vi "FPGA_HoppingStep(NoXYCalculation).vi"() -> ()   [LabVIEW 2014]
uses:
  <vilib>/rvi/Emulation/niFpgaGetClockAttributes.vi
  <vilib>/rvi/Emulation/niFpgaSctlEmulationGetInTimedLoop.vi
  <vilib>/rvi/Emulation/niFpgaEmulationReportErrorSimple.vi
  <vilib>/rvi/interface/RandomDataEmulation/niFpgaRandomDataHandleErrors.vi
  <vilib>/rvi/eio/common/nirviEmuTemplateMethod_errors.vi
  <vilib>/rvi/Emulation/niFpgaProcessEmulError.vi
  <vilib>/rvi/Emulation/niFpgaCriticalErrorInLSC.vi
  <vilib>/rvi/DataTransferAndStorage/Container/XNode/niFpgaContainer.xnode
  <vilib>/rvi/interface/RandomDataEmulation/nirviRandomDataFpgaReadWriteTemplate.vi
  <vilib>/eio/EIONode/EIONode.xnode
panel:
  out "ZPresPos":i16
  in  "stop":bool
  in  "Sleep us":i16
  in  "RelativeWithdraw":i16
  in  "ZOffset":i16
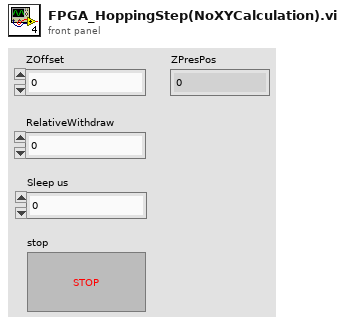
[diagram p1: front panel]
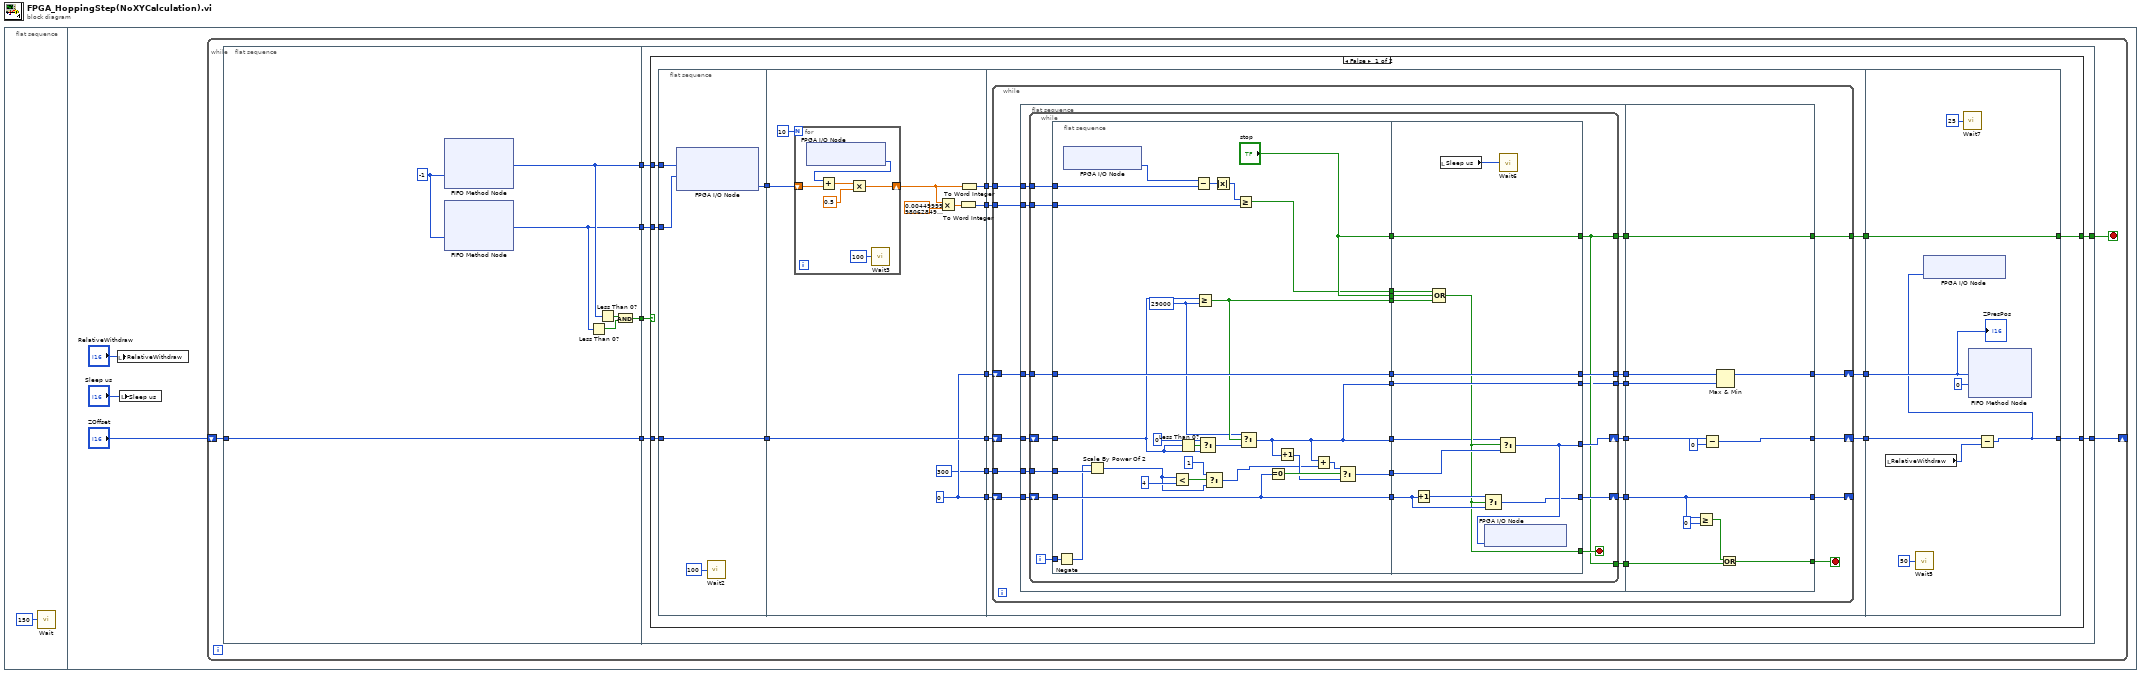
[diagram p0: block diagram]
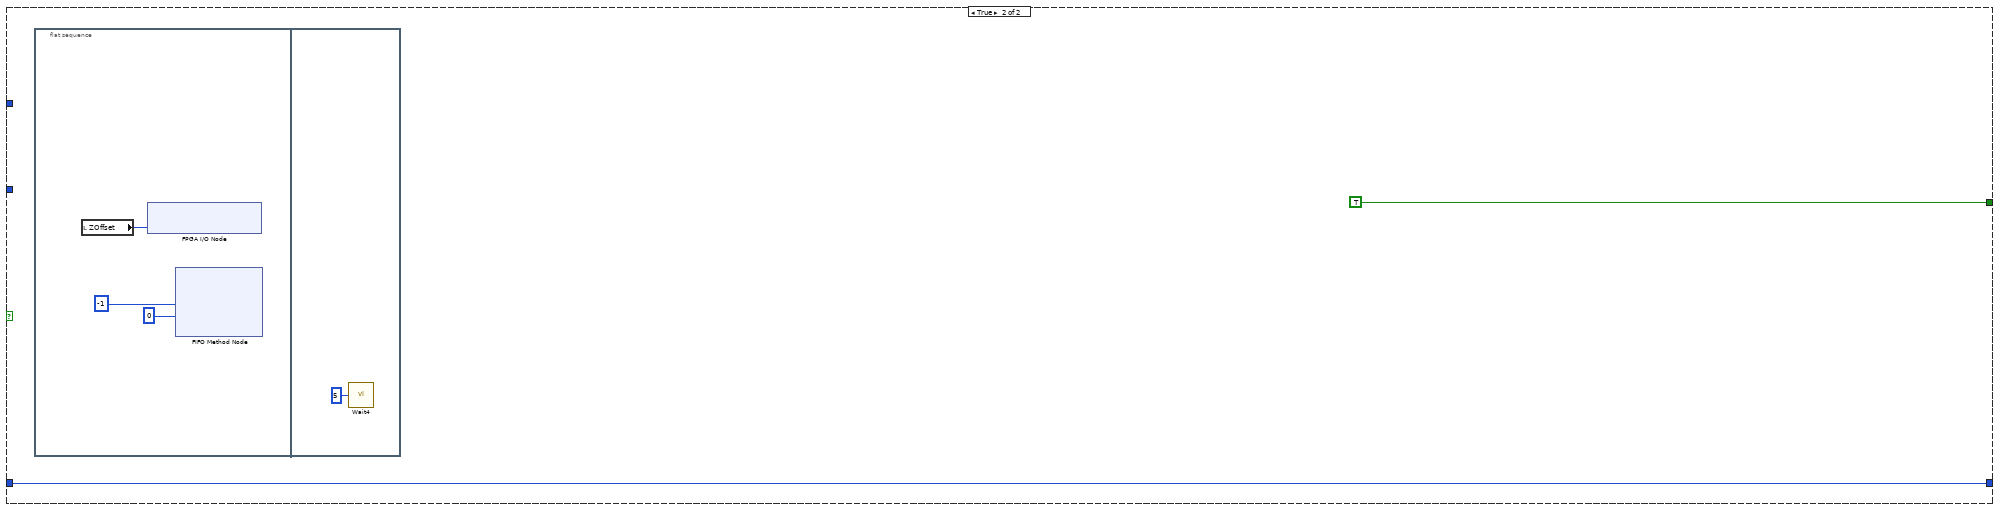
[diagram p2: hidden frame]
diagram:
  n1 = flat-sequence {
    frame #0 {
      n2 = call "Wait"("Count(mSec)"=u32 150) -> ()  [unwired: 1 out]
    }
    frame #1 {
      n3 = local write "RelativeWithdraw"("RelativeWithdraw") -> ()
      n4 = local write "Sleep us"("Sleep us") -> ()
      n5 = while {
        shift-right: [w6] -> _
        shift-left: "ZOffset" -> [w8]
        stop <- w5 stop-if-true
        n6 = flat-sequence {
          tunnel: [w18] -> w11
          tunnel: [w17] -> w10
          tunnel: [w14] -> w9
          tunnel: w8 -> [w13]
          tunnel: [w13] -> w7
          tunnel: w11 -> [w24]
          tunnel: w10 -> [w23]
          tunnel: w9 -> [w22]
          tunnel: w7 -> [w21]
          tunnel: [w20] -> w6
          tunnel: [w19] -> w5
          frame #0 {
            w12 = -1 ("Timeout")
            n7 = xnode ("FIFO Method Node")("Timeout"=w12) -> ("Element"=w18:i16)  [unwired: 1 in, 2 out]
            n8 = xnode ("FIFO Method Node")("Timeout"=w12) -> ("Element"=w17:i16)  [unwired: 1 in, 2 out]
            n9 = Less Than 0?(x=w17) -> (x < 0?=w15:bool)
            n10 = Less Than 0?(x=w18) -> (x < 0?=w16:bool)
            n11 = And(x=w16, y=w15) -> (x .and. y?=w14:bool)
          }
          frame #1 {
            n12 = case shown="False" w22 {
              tunnel: w24 -> [w40 _]
              tunnel: w23 -> [w39 _]
              tunnel: w21 -> [w38 w184]
              tunnel: [w28 TRUE ("stop")] -> w19
              tunnel: [w27 w184] -> w20
              frame False {
                n13 = flat-sequence {
                  tunnel: w40 -> [w45]
                  tunnel: w39 -> [w44]
                  tunnel: w38 -> [w42]
                  tunnel: [w42] -> w37
                  tunnel: [w41] -> w35
                  tunnel: w37 -> [w55]
                  tunnel: [w55] -> w36
                  tunnel: w35 -> [w54]
                  tunnel: [w47] -> w34
                  tunnel: [w49] -> w33
                  tunnel: [w48] -> w32
                  tunnel: [w47] -> w31
                  tunnel: [i16 300] -> w25
                  tunnel: w36 -> [w70]
                  tunnel: w34 -> [w67]
                  tunnel: w33 -> [w69]
                  tunnel: w32 -> [w68]
                  tunnel: w31 -> [w66]
                  tunnel: [w65] -> w30
                  tunnel: [w64] -> w29
                  tunnel: [w63] -> w26
                  tunnel: w25 -> [w62]
                  tunnel: w30 -> [w180]
                  tunnel: w29 -> [w183]
                  tunnel: [w183] -> w28
                  tunnel: [w177] -> w27
                  tunnel: w26 -> [w179]
                  frame #0 {
                    n14 = xnode "FPGA I/O Node"("Connector0/AO2"=w45, "Connector0/AO3"=w44) -> ("Connector0/AI1"=w41:i16)  [unwired: 3 in, 3 out]
                    n15 = call "Wait2"("Count(uSec)"=u32 100) -> ()  [unwired: 1 out]
                  }
                  frame #1 {
                    w47 = i16 0
                    n16 = for {
                      N: 10 -> [_]
                      shift-right: [w56] -> w50
                      shift-left: w54 -> [w60]
                      n17 = xnode "FPGA I/O Node"() -> ("Connector0/AI1"=w59:i16)  [unwired: 1 in, 1 out]
                      n18 = Add(x=w59, y=w60) -> (x+y=w58:sgl)
                      n19 = Multiply(x=w58, y=sgl 0.5) -> (x*y=w56:sgl)
                      n20 = call "Wait3"("Count(uSec)"=u32 100) -> ()  [unwired: 1 out]
                    }
                    n21 = Multiply(x=w50, y=sgl 0.0045) -> (x*y=w51:sgl)
                    n22 = To Word Integer(number=w51) -> (16bit integer=w48:i16)
                    n23 = To Word Integer(number=w50) -> (16bit integer=w49:i16)
                  }
                  frame #2 {
                    n24 = while {
                      tunnel: w69 -> [w84]
                      tunnel: w68 -> [w83]
                      tunnel: [w79] -> w64
                      shift-right: [w80] -> w65
                      shift-left: w66 -> [w81]
                      shift-right: [w73] -> w63
                      shift-left: w70 -> [w85]
                      shift-right: [w72] -> _
                      shift-left: w67 -> [w82]
                      tunnel: w62 -> [w71]
                      stop <- w76 stop-if-true
                      n25 = flat-sequence {
                        tunnel: w85 -> [w99]
                        tunnel: w84 -> [w98]
                        tunnel: w83 -> [w97]
                        tunnel: w82 -> [w96]
                        tunnel: w81 -> [w95]
                        tunnel: [w94] -> w87
                        tunnel: [w93] -> w86
                        tunnel: [w92] -> w78
                        tunnel: [w91] -> w77
                        tunnel: [w90] -> w75
                        tunnel: [w89] -> w74
                        tunnel: w71 -> [w88]
                        tunnel: [w175] -> w79
                        tunnel: [w169] -> w80
                        tunnel: w87 -> [w170]
                        tunnel: w86 -> [w175]
                        tunnel: w78 -> [w167]
                        tunnel: w77 -> [w173]
                        tunnel: [w171] -> w76
                        tunnel: w75 -> [w168]
                        tunnel: w74 -> [w166]
                        tunnel: [w164] -> w73
                        tunnel: [w167] -> w72
                        frame #0 {
                          n26 = while {
                            tunnel: w98 -> [w120]
                            tunnel: w97 -> [w119]
                            shift-right: [w117] -> w92
                            shift-left: w96 -> [w118]
                            shift-right: [w116] -> w89
                            shift-left: w99 -> [w121]
                            tunnel: [w105] -> w93
                            tunnel: w95 -> [w115]
                            tunnel: [w113] -> w94
                            tunnel: [w105] -> w91
                            tunnel: [w104] -> w90
                            tunnel: w88 -> [w102]
                            i -> [w101]
                            stop <- w106 stop-if-true
                            n27 = flat-sequence {
                              tunnel: [w149] -> w114
                              tunnel: [w140] -> w112
                              tunnel: ["stop"] -> w111
                              tunnel: [w140] -> w110
                              tunnel: [w146] -> w109
                              tunnel: ["stop"] -> w108
                              tunnel: [w147] -> w107
                              tunnel: [w145] -> w103
                              tunnel: [w142] -> w100
                              tunnel: w101 -> [w127]
                              tunnel: w102 -> [w128]
                              tunnel: w115 -> [w149]
                              tunnel: w118 -> [w145]
                              tunnel: w119 -> [w134]
                              tunnel: w120 -> [w137]
                              tunnel: w121 -> [w130]
                              tunnel: [w162] -> w116
                              tunnel: [w154] -> w117
                              tunnel: w114 -> [w158]
                              tunnel: [w158] -> w113
                              tunnel: [w151] -> w106
                              tunnel: w112 -> [w157]
                              tunnel: [w163] -> w105
                              tunnel: w111 -> [w163]
                              tunnel: w110 -> [w150]
                              tunnel: w109 -> [w159]
                              tunnel: w108 -> [w161]
                              tunnel: w107 -> [w160]
                              tunnel: [w157] -> w104
                              tunnel: w103 -> [w155]
                              tunnel: w100 -> [w152]
                              frame #0 {
                                w133 = i16 29000 ("y")
                                n28 = Negate(x=w127) -> (-x=w126:i32)
                                n29 = xnode "FPGA I/O Node"() -> ("Connector0/AI1"=w138:i16)  [unwired: 1 in, 1 out]
                                n30 = Scale By Power Of 2(n=w126, x=w128) -> (x*2^n=w122:i16)
                                n31 = Less?(x=w122, y=i16 4) -> (x < y?=w124:bool)
                                n32 = Less Than 0?(x=w130) -> (x < 0?=w131:bool)
                                n33 = Subtract(x=w138, y=w137) -> (x-y=w136:i16)
                                n34 = Greater Or Equal?(x=w130, y=w133) -> (x >= y?=w147:bool)
                                n35 = Select(t=i16 0, s=w131, f=w130) -> (s? t:f=w129:i16)
                                n36 = Select(t=i16 1 ("y"), s=w124, f=w122) -> (s? t:f=w141:i16)
                                n37 = Absolute Value(x=w136) -> (abs(x)=w135:i16)
                                n38 = Greater Or Equal?(x=w135, y=w134) -> (x >= y?=w146:bool)
                                n39 = Select(t=w133, s=w147, f=w129) -> (s? t:f=w140:i16)
                                n40 = Equal To 0?(x=w145) -> (x = 0?=w144:bool)
                                n41 = Increment(x=w140) -> (x+1=w143:i16)
                                n42 = Add(x=w140, y=w141) -> (x+y=w139:i16)
                                n43 = Select(t=w139, s=w144, f=w143) -> (s? t:f=w142:i16)
                              }
                              frame #1 {
                                n44 = Increment(x=w155) -> (x+1=w156:i16)
                                n45 = Compound Arithmetic op=OR(w159, w161, w160) -> (w151:bool)
                                n46 = local read "Sleep us"() -> (w153:i16)
                                n47 = Select(t=w156, s=w151, f=w155) -> (s? t:f=w154:i16)
                                n48 = Select(t=w150, s=w151, f=w152) -> (s? t:f=w162:i16)
                                n49 = xnode "FPGA I/O Node"("Connector0/AO0"=w162) -> ()  [unwired: 1 in, 1 out]
                                n50 = call "Wait6"("Count(uSec)"=w153) -> ()  [unwired: 1 out]
                              }
                            }
                          }
                        }
                        frame #1 {
                          n51 = Greater Or Equal?(x=w167, y=i16 0) -> (x >= y?=w172:bool)
                          n52 = Subtract(x=w166, y=i16 0) -> (x-y=w164:i16)
                          n53 = Max & Min(x=w170, y=w168) -> (max(x,y)=w169:i16)  [unwired: 1 out]
                          n54 = Or(x=w172, y=w173) -> (x .or. y?=w171:bool)
                        }
                      }
                    }
                  }
                  frame #3 {
                    n55 = local read "RelativeWithdraw"() -> (w178:i16)
                    n56 = call "Wait5"("Count(uSec)"=u32 50) -> ()  [unwired: 1 out]
                    n57 = call "Wait7"("Count(uSec)"=u32 25) -> ()  [unwired: 1 out]
                    n58 = xnode ("FIFO Method Node")("Element"=w180, "Timeout"=0) -> ()  [unwired: 1 in, 2 out]
                    n59 = Subtract(x=w179, y=w178) -> (x-y=w177:i16)
                    n60 = xnode "FPGA I/O Node"("Connector0/AO0"=w177) -> ()  [unwired: 1 in, 1 out]
                    "ZPresPos" <- w180
                  }
                }
              }
              frame True {
                n61 = flat-sequence {
                  frame #0 {
                    n62 = local read "ZOffset"() -> (w188:i16)
                    n63 = xnode "FPGA I/O Node"("Connector0/AO0"=w188) -> ()  [unwired: 1 in, 1 out]
                    n64 = xnode ("FIFO Method Node")("Element"=i16 -1, "Timeout"=0) -> ()  [unwired: 1 in, 2 out]
                  }
                  frame #1 {
                    n65 = call "Wait4"("Count(mSec)"=u32 5) -> ()  [unwired: 1 out]
                  }
                }
              }
            }
          }
        }
      }
    }
  }
